vi "首页.vi"() -> ()   [LabVIEW 2016]
uses:
  <vilib>/Utility/miscctls.llb/LVPointTypeDef.ctl
  <vilib>/Utility/sysdir.llb/System Directory Type.ctl
  <vilib>/addons/database/_DB Variant To Data/Database Variant To Data.xnode
panel:
  out "显示":T1
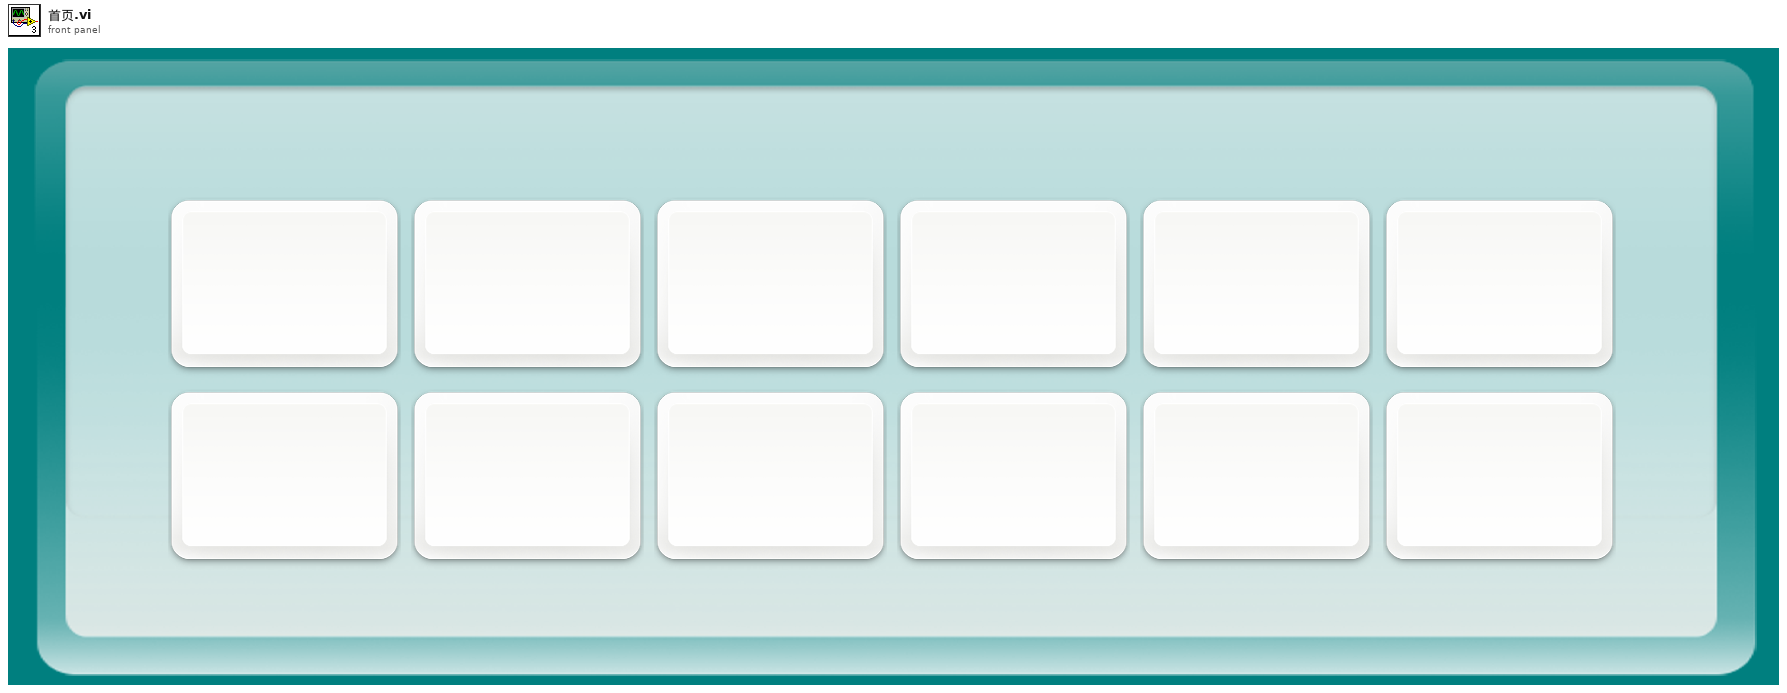
[diagram p1: front panel]
types:
  T1 = typedef "多数值显示.ctl" = cluster{"显示":T2, "显示 2":T2, "显示 3":T2, "显示 4":T2, "显示 5":T2, "显示 6":T2, "显示 12":T2, "显示 11":T2, "显示 10":T2, "显示 9":T2, "显示 8":T2, "显示 7":T2}
  T2 = typedef "数值显示.ctl" = cluster{"中文项目名称":string, "英文项目名称":string, "浓度":string, "单位":string}
  T3 = typedef "LVPointTypeDef.ctl" = cluster{"Horizontal":i16, "Vertical":i16}
  T4 = cluster{"显示参数中文名":string, "显示参数英文名":string, "显示浓度":string, "显示单位":string}[]
  T5 = cluster{"显示参数中文名":string, "显示参数英文名":string, "显示浓度":string, "显示单位":string}
  T6 = typedef "System Directory Type.ctl" = i32
  T7 = cluster{"AD0":dbl, "AD1":dbl, "AD2":dbl, "AD3":dbl, "AD4":dbl, "AD5":dbl, "AD6":dbl, "AD7":dbl}
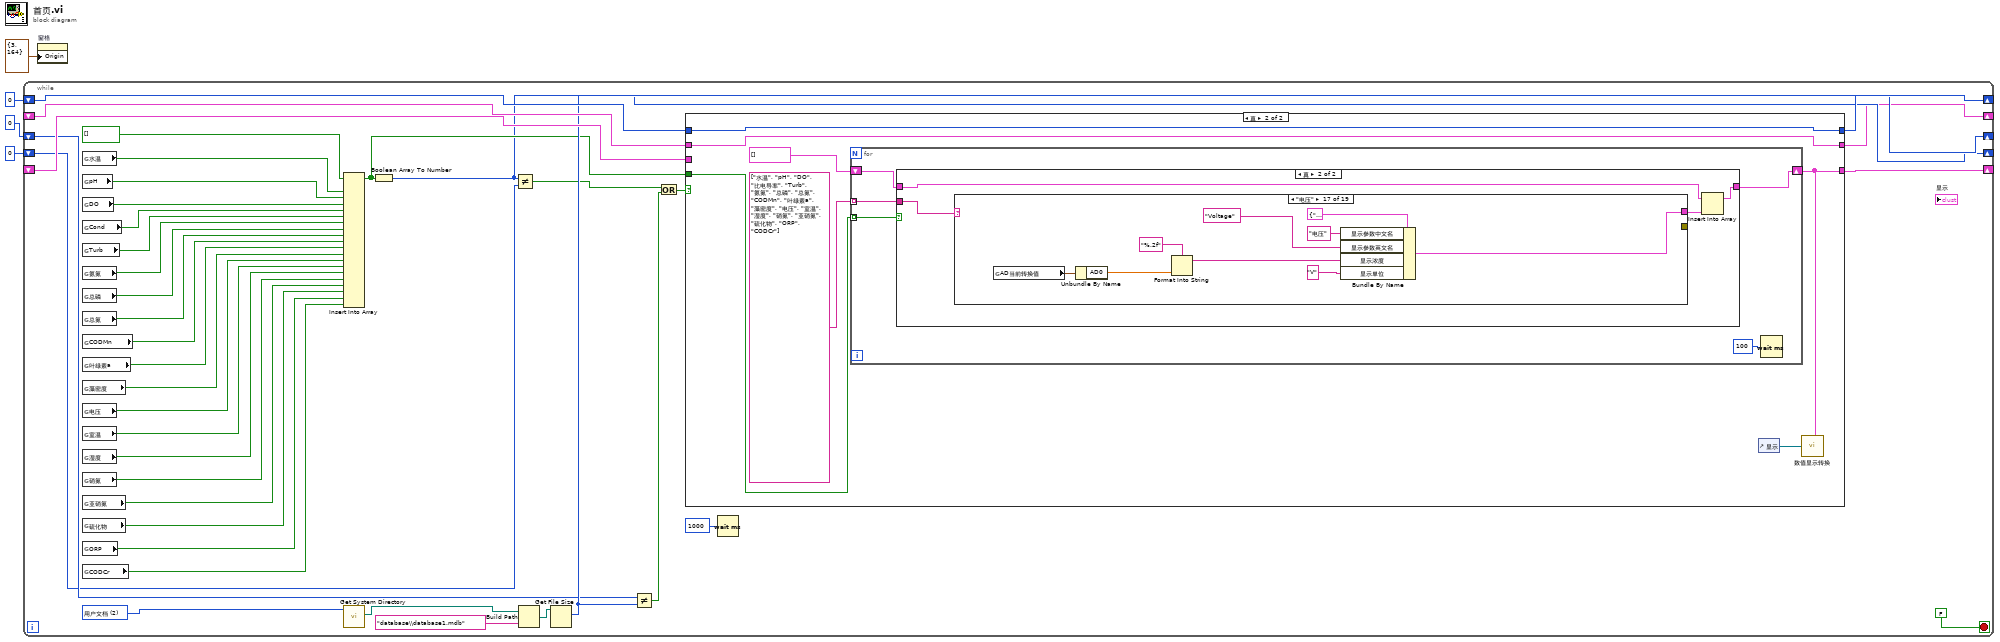
[diagram p0: block diagram]
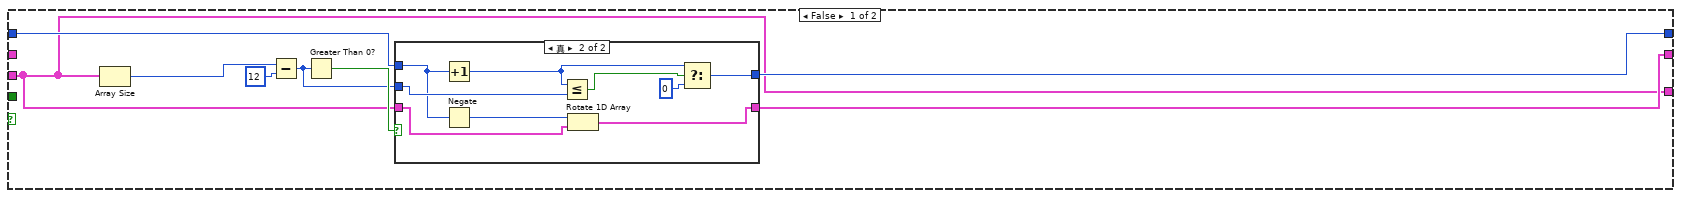
[diagram p2: hidden frame]
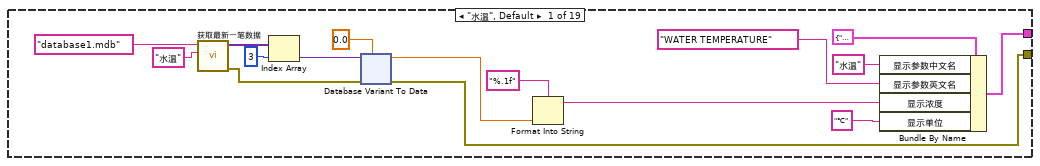
[diagram p5: hidden frame]
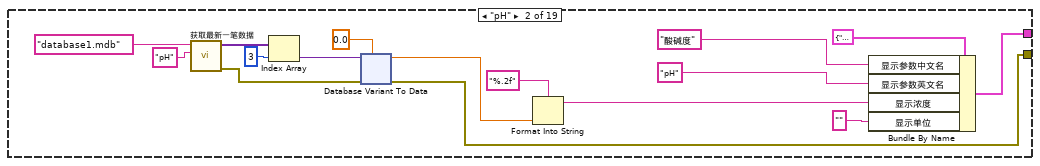
[diagram p6: hidden frame]
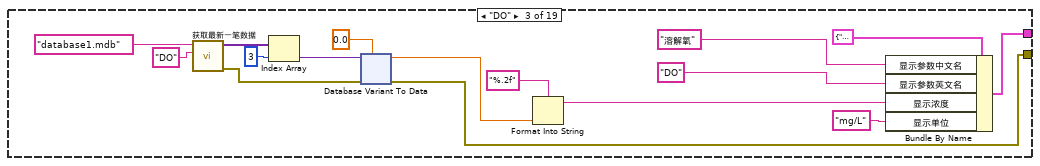
[diagram p7: hidden frame]
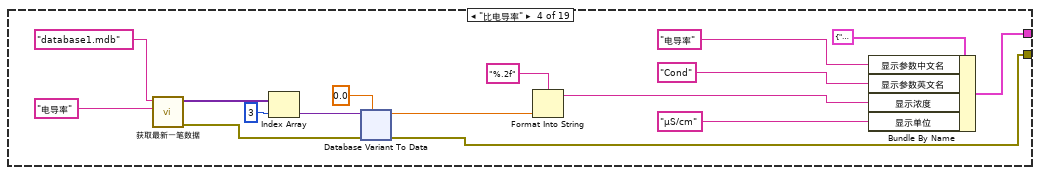
[diagram p8: hidden frame]
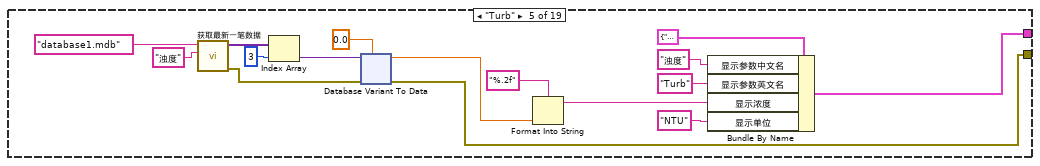
[diagram p9: hidden frame]
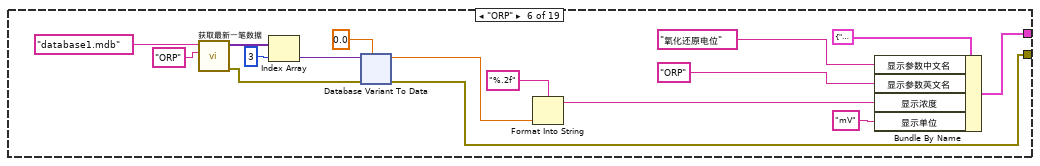
[diagram p10: hidden frame]
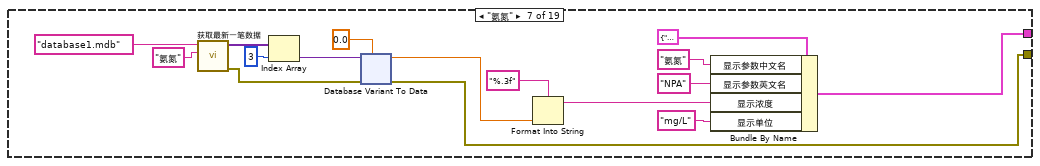
[diagram p11: hidden frame]
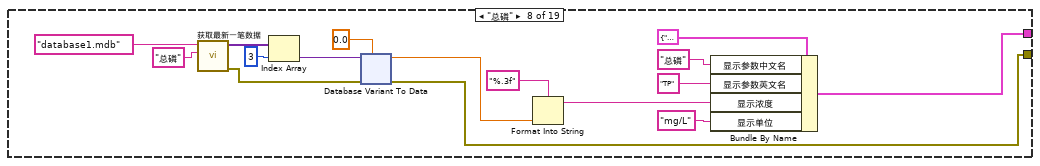
[diagram p12: hidden frame]
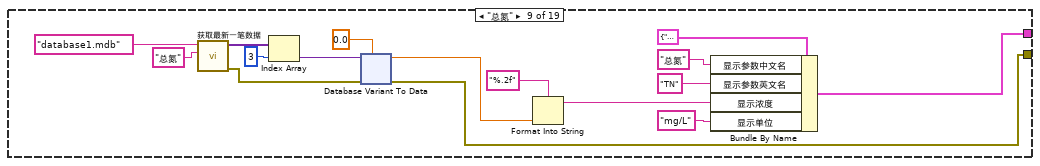
[diagram p13: hidden frame]
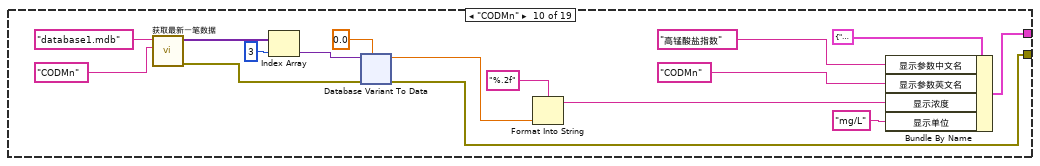
[diagram p14: hidden frame]
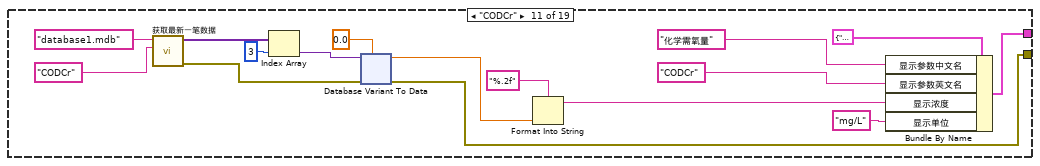
[diagram p15: hidden frame]
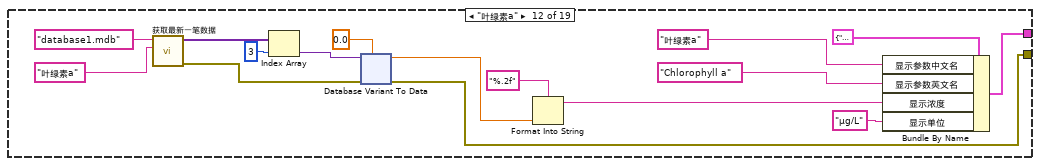
[diagram p16: hidden frame]
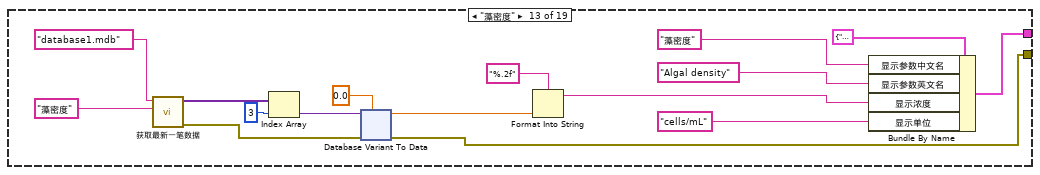
[diagram p17: hidden frame]
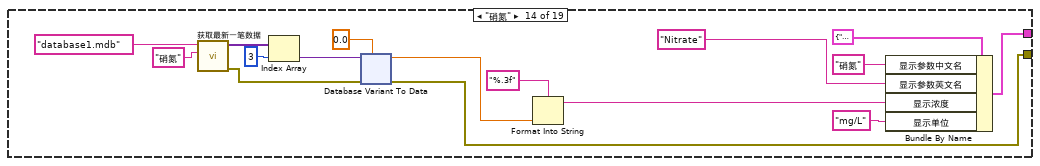
[diagram p18: hidden frame]
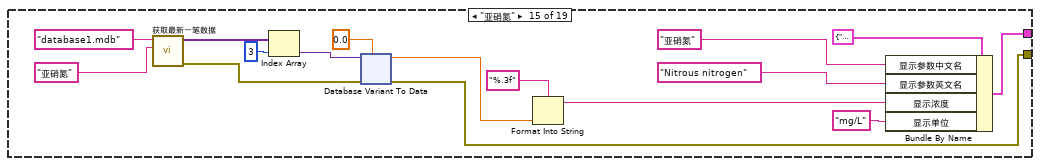
[diagram p19: hidden frame]
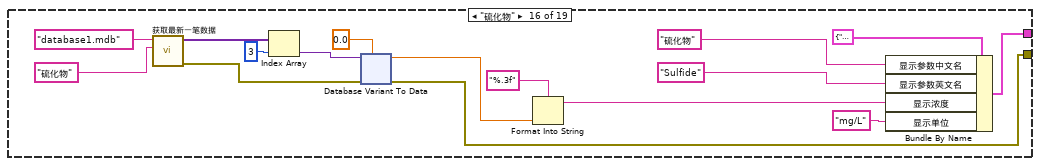
[diagram p20: hidden frame]
diagram:
  n1 = while {
    shift-right: [w42] -> _
    shift-left: _ -> [w41]
    shift-right: [w40] -> _
    shift-left: 0 -> [w43]
    shift-right: [w5] -> _
    shift-left: _ -> [w39]
    shift-right: [w34] -> _
    shift-left: i64 0 ("size (in bytes)") -> [w33]
    shift-right: [w12] -> _
    shift-left: u32 0 -> [w11]
    stop <- FALSE stop-if-true
    w38 = T6 2 items=["用户目录"=0, "用户桌面"=1, "用户文档"=2, "用户应用程序数据"=3, "用户设置"=4, "用户临时目录"=5, "公共文档"=6, "公共应用程序数据"=7, "公共设置"=8, "公共缓存"=13, "系统核心库"=9, "系统安装库"=10, "应用程序文件"=11, "启动盘根目录"=12] ("system directory type")
    n2 = global read "首页设置全局变量.vi" "水温"() -> (w26:bool)
    n3 = global read "首页设置全局变量.vi" "pH"() -> (w25:bool)
    n4 = global read "首页设置全局变量.vi" "DO"() -> (w24:bool)
    n5 = global read "首页设置全局变量.vi" "Cond"() -> (w23:bool)
    n6 = global read "首页设置全局变量.vi" "Turb"() -> (w22:bool)
    n7 = global read "首页设置全局变量.vi" "氨氮"() -> (w21:bool)
    n8 = global read "首页设置全局变量.vi" "总磷"() -> (w20:bool)
    n9 = global read "首页设置全局变量.vi" "总氮"() -> (w19:bool)
    n10 = global read "首页设置全局变量.vi" "CODMn"() -> (w18:bool)
    n11 = global read "首页设置全局变量.vi" "叶绿素a"() -> (w17:bool)
    n12 = global read "首页设置全局变量.vi" "藻密度"() -> (w16:bool)
    n13 = global read "首页设置全局变量.vi" "电压"() -> (w15:bool)
    n14 = global read "首页设置全局变量.vi" "室温"() -> (w14:bool)
    n15 = global read "首页设置全局变量.vi" "湿度"() -> (w28:bool)
    n16 = global read "首页设置全局变量.vi" "硝氮"() -> (w29:bool)
    n17 = global read "首页设置全局变量.vi" "亚硝氮"() -> (w30:bool)
    n18 = global read "首页设置全局变量.vi" "硫化物"() -> (w31:bool)
    n19 = global read "首页设置全局变量.vi" "ORP"() -> (w32:bool)
    n20 = global read "首页设置全局变量.vi" "CODCr"() -> (w6:bool)
    n21 = Insert Into Array(array=bool[] [], new element #1=w26, new element #2=w25, new element #3=w24, new element #4=w23, new element #5=w22, new element #6=w21, new element #7=w20, new element #8=w19, new element #9=w18, new element #10=w17, new element #11=w16, new element #12=w15, new element #13=w14, new element #14=w28, new element #15=w29, new element #16=w30, new element #17=w31, new element #18=w32, new element #19=w6) -> (w13:bool[])  [unwired: 1 in]
    n22 = call <vilib>:"Get System Directory.vi"("system directory type"=w38) -> ("system directory"=w37:path)  [unwired: 10 in]
    n23 = Boolean Array To Number(Boolean array=w13) -> (number=w12:u32)
    n24 = Not Equal?(x=w12, y=w11) -> (x != y?=w10:bool)
    n25 = Build Path(base path=w37, name or relative path="database\\database1.mdb" ("名称或相对路径")) -> (appended path=w35:path)
    n26 = Get File Size(file=w35) -> (size (in bytes)=w34:i64)  [unwired: 1 in, 2 out]
    n27 = Not Equal?(x=w33, y=w34) -> (x != y?=w9:bool)
    n28 = Or(x=w10, y=w9) -> (x .or. y?=w8:bool)
    n29 = case shown="真" w8 {
      tunnel: w43 -> [w52 w67]
      tunnel: [w45 w63] -> w42
      tunnel: w41 -> [w45 _]
      tunnel: [w51 w67] -> w40
      tunnel: [w46 w66] -> w5
      tunnel: w39 -> [_ w66]
      tunnel: w13 -> [_ w65]
      frame False {
        n30 = Array Size(array=w45) -> (size(s)=w50:i32)
        n31 = Subtract(x=w50, y=12) -> (x-y=w47:i32)
        n32 = Greater Than 0?(x=w47) -> (x > 0?=w48:bool)
        n33 = case shown="真" w48 {
          tunnel: w45 -> [w53 w62]
          tunnel: w52 -> [_ w55]
          tunnel: [w53 w61] -> w46
          tunnel: [_ w56] -> w51
          tunnel: w47 -> [_ w59]
          frame False {
          }
          frame True {
            n34 = Increment(x=w55) -> (x+1=w60:i32)
            n35 = Negate(x=w55) -> (-x=w54:i32)
            n36 = Less Or Equal?(x=w60, y=w59) -> (x <= y?=w58:bool)
            n37 = Rotate 1D Array(1:w62, 2:w54) -> (0:w61:T4)
            n38 = Select(t=w60, s=w58, f=0) -> (s? t:f=w56:i32)
          }
        }
      }
      frame True {
        n39 = for {
          tunnel: w65 -> [w74] mode=indexing
          tunnel: string[] ["水温", "pH", "DO", "比电导率", "Turb", "氨氮", "总磷", "总氮", "CODMn", "叶绿素a", "藻密度", "电压", "室温", "湿度", "硝氮", "亚硝氮", "硫化物", "ORP", "CODCr"] -> [w73] mode=indexing
          shift-right: [w71] -> w63
          shift-left: T4 [] -> [w72]
          n40 = case shown="真" w74 {
            tunnel: w73 -> [_ w79]
            tunnel: w72 -> [w75 w78]
            tunnel: [w75 w77] -> w71
            frame False {
            }
            frame True {
              n41 = case shown="\"电压\"" w79 {
                tunnel: [w89 w139 w187 w235 w283 w331 w379 w427 w475 w523 w571 w619 w667 w715 w763 w811 w852 w861 w870] -> w76
                tunnel: [w88 w136 w184 w231 w279 w327 w368 w416 w464 w512 w560 w615 w656 w704 w752 w800 _ _ _] -> _
                frame "水温", Default {
                  n42 = call "获取最新一笔数据.vi"("table"="水温", "database"="database1.mdb" ("名称或相对路径")) -> ("error out"=w80:errorcluster, "子数组"=w85:variant[])  [unwired: 8 in]
                  n43 = Index Array(array=w85, index=3 ("索引")) -> (element=w83:variant)
                  n44 = xnode "Database Variant To Data"("database variant"=w83, "error in (no error)"=w80, "type"=0.0) -> ("data"=w87:dbl, "error out"=w88:errorcluster)
                  n45 = Format Into String(format string="%.1f" ("格式字符串"), w87) -> (resulting string=w90:string)  [unwired: 2 in, 1 out]
                  n46 = Bundle By Name(cluster=T5 {"显示参数中文名"="", "显示参数英文名"="", "显示浓度"="", "显示单位"=""} ("元素"), "显示参数中文名"="水温", "显示参数英文名"="WATER TEMPERATURE", "显示浓度"=w90, "显示单位"="℃") -> (w89:T5)
                }
                frame "pH" {
                  n47 = call "获取最新一笔数据.vi"("table"="pH", "database"="database1.mdb" ("名称或相对路径")) -> ("error out"=w128:errorcluster, "子数组"=w133:variant[])  [unwired: 8 in]
                  n48 = Index Array(array=w133, index=3 ("索引")) -> (element=w131:variant)
                  n49 = xnode "Database Variant To Data"("database variant"=w131, "error in (no error)"=w128, "type"=0.0) -> ("data"=w135:dbl, "error out"=w136:errorcluster)
                  n50 = Format Into String(format string="%.2f" ("格式字符串"), w135) -> (resulting string=w137:string)  [unwired: 2 in, 1 out]
                  n51 = Bundle By Name(cluster=T5 {"显示参数中文名"="", "显示参数英文名"="", "显示浓度"="", "显示单位"=""} ("元素"), "显示参数中文名"="酸碱度", "显示参数英文名"="pH", "显示浓度"=w137, "显示单位"="") -> (w139:T5)
                }
                frame "DO" {
                  n52 = call "获取最新一笔数据.vi"("table"="DO", "database"="database1.mdb" ("名称或相对路径")) -> ("error out"=w176:errorcluster, "子数组"=w181:variant[])  [unwired: 8 in]
                  n53 = Index Array(array=w181, index=3 ("索引")) -> (element=w179:variant)
                  n54 = xnode "Database Variant To Data"("database variant"=w179, "error in (no error)"=w176, "type"=0.0) -> ("data"=w183:dbl, "error out"=w184:errorcluster)
                  n55 = Format Into String(format string="%.2f" ("格式字符串"), w183) -> (resulting string=w185:string)  [unwired: 2 in, 1 out]
                  n56 = Bundle By Name(cluster=T5 {"显示参数中文名"="", "显示参数英文名"="", "显示浓度"="", "显示单位"=""} ("元素"), "显示参数中文名"="溶解氧", "显示参数英文名"="DO", "显示浓度"=w185, "显示单位"="mg/L") -> (w187:T5)
                }
                frame "比电导率" {
                  n57 = call "获取最新一笔数据.vi"("table"="电导率", "database"="database1.mdb" ("名称或相对路径")) -> ("error out"=w224:errorcluster, "子数组"=w229:variant[])  [unwired: 8 in]
                  n58 = Index Array(array=w229, index=3 ("索引")) -> (element=w227:variant)
                  n59 = xnode "Database Variant To Data"("database variant"=w227, "error in (no error)"=w224, "type"=0.0) -> ("data"=w232:dbl, "error out"=w231:errorcluster)
                  n60 = Format Into String(format string="%.2f" ("格式字符串"), w232) -> (resulting string=w233:string)  [unwired: 2 in, 1 out]
                  n61 = Bundle By Name(cluster=T5 {"显示参数中文名"="", "显示参数英文名"="", "显示浓度"="", "显示单位"=""} ("元素"), "显示参数中文名"="电导率", "显示参数英文名"="Cond", "显示浓度"=w233, "显示单位"="μS/cm") -> (w235:T5)
                }
                frame "Turb" {
                  n62 = call "获取最新一笔数据.vi"("table"="浊度", "database"="database1.mdb" ("名称或相对路径")) -> ("error out"=w272:errorcluster, "子数组"=w277:variant[])  [unwired: 8 in]
                  n63 = Index Array(array=w277, index=3 ("索引")) -> (element=w275:variant)
                  n64 = xnode "Database Variant To Data"("database variant"=w275, "error in (no error)"=w272, "type"=0.0) -> ("data"=w280:dbl, "error out"=w279:errorcluster)
                  n65 = Format Into String(format string="%.2f" ("格式字符串"), w280) -> (resulting string=w281:string)  [unwired: 2 in, 1 out]
                  n66 = Bundle By Name(cluster=T5 {"显示参数中文名"="", "显示参数英文名"="", "显示浓度"="", "显示单位"=""} ("元素"), "显示参数中文名"="浊度", "显示参数英文名"="Turb", "显示浓度"=w281, "显示单位"="NTU") -> (w283:T5)
                }
                frame "ORP" {
                  n67 = call "获取最新一笔数据.vi"("table"="ORP", "database"="database1.mdb" ("名称或相对路径")) -> ("error out"=w320:errorcluster, "子数组"=w325:variant[])  [unwired: 8 in]
                  n68 = Index Array(array=w325, index=3 ("索引")) -> (element=w323:variant)
                  n69 = xnode "Database Variant To Data"("database variant"=w323, "error in (no error)"=w320, "type"=0.0) -> ("data"=w328:dbl, "error out"=w327:errorcluster)
                  n70 = Format Into String(format string="%.2f" ("格式字符串"), w328) -> (resulting string=w329:string)  [unwired: 2 in, 1 out]
                  n71 = Bundle By Name(cluster=T5 {"显示参数中文名"="", "显示参数英文名"="", "显示浓度"="", "显示单位"=""} ("元素"), "显示参数中文名"="氧化还原电位", "显示参数英文名"="ORP", "显示浓度"=w329, "显示单位"="mV") -> (w331:T5)
                }
                frame "氨氮" {
                  n72 = call "获取最新一笔数据.vi"("table"="氨氮", "database"="database1.mdb" ("名称或相对路径")) -> ("error out"=w369:errorcluster, "子数组"=w375:variant[])  [unwired: 8 in]
                  n73 = Index Array(array=w375, index=3 ("索引")) -> (element=w373:variant)
                  n74 = xnode "Database Variant To Data"("database variant"=w373, "error in (no error)"=w369, "type"=0.0) -> ("data"=w370:dbl, "error out"=w368:errorcluster)
                  n75 = Format Into String(format string="%.3f" ("格式字符串"), w370) -> (resulting string=w377:string)  [unwired: 2 in, 1 out]
                  n76 = Bundle By Name(cluster=T5 {"显示参数中文名"="", "显示参数英文名"="", "显示浓度"="", "显示单位"=""} ("元素"), "显示参数中文名"="氨氮", "显示参数英文名"="NPA", "显示浓度"=w377, "显示单位"="mg/L") -> (w379:T5)
                }
                frame "总磷" {
                  n77 = call "获取最新一笔数据.vi"("table"="总磷", "database"="database1.mdb" ("名称或相对路径")) -> ("error out"=w417:errorcluster, "子数组"=w423:variant[])  [unwired: 8 in]
                  n78 = Index Array(array=w423, index=3 ("索引")) -> (element=w421:variant)
                  n79 = xnode "Database Variant To Data"("database variant"=w421, "error in (no error)"=w417, "type"=0.0) -> ("data"=w418:dbl, "error out"=w416:errorcluster)
                  n80 = Format Into String(format string="%.3f" ("格式字符串"), w418) -> (resulting string=w425:string)  [unwired: 2 in, 1 out]
                  n81 = Bundle By Name(cluster=T5 {"显示参数中文名"="", "显示参数英文名"="", "显示浓度"="", "显示单位"=""} ("元素"), "显示参数中文名"="总磷", "显示参数英文名"="TP", "显示浓度"=w425, "显示单位"="mg/L") -> (w427:T5)
                }
                frame "总氮" {
                  n82 = call "获取最新一笔数据.vi"("table"="总氮", "database"="database1.mdb" ("名称或相对路径")) -> ("error out"=w465:errorcluster, "子数组"=w471:variant[])  [unwired: 8 in]
                  n83 = Index Array(array=w471, index=3 ("索引")) -> (element=w469:variant)
                  n84 = xnode "Database Variant To Data"("database variant"=w469, "error in (no error)"=w465, "type"=0.0) -> ("data"=w466:dbl, "error out"=w464:errorcluster)
                  n85 = Format Into String(format string="%.2f" ("格式字符串"), w466) -> (resulting string=w473:string)  [unwired: 2 in, 1 out]
                  n86 = Bundle By Name(cluster=T5 {"显示参数中文名"="", "显示参数英文名"="", "显示浓度"="", "显示单位"=""} ("元素"), "显示参数中文名"="总氮", "显示参数英文名"="TN", "显示浓度"=w473, "显示单位"="mg/L") -> (w475:T5)
                }
                frame "CODMn" {
                  n87 = call "获取最新一笔数据.vi"("table"="CODMn", "database"="database1.mdb" ("名称或相对路径")) -> ("error out"=w513:errorcluster, "子数组"=w519:variant[])  [unwired: 8 in]
                  n88 = Index Array(array=w519, index=3 ("索引")) -> (element=w517:variant)
                  n89 = xnode "Database Variant To Data"("database variant"=w517, "error in (no error)"=w513, "type"=0.0) -> ("data"=w514:dbl, "error out"=w512:errorcluster)
                  n90 = Format Into String(format string="%.2f" ("格式字符串"), w514) -> (resulting string=w521:string)  [unwired: 2 in, 1 out]
                  n91 = Bundle By Name(cluster=T5 {"显示参数中文名"="", "显示参数英文名"="", "显示浓度"="", "显示单位"=""} ("元素"), "显示参数中文名"="高锰酸盐指数", "显示参数英文名"="CODMn", "显示浓度"=w521, "显示单位"="mg/L") -> (w523:T5)
                }
                frame "CODCr" {
                  n92 = call "获取最新一笔数据.vi"("table"="CODCr", "database"="database1.mdb" ("名称或相对路径")) -> ("error out"=w561:errorcluster, "子数组"=w567:variant[])  [unwired: 8 in]
                  n93 = Index Array(array=w567, index=3 ("索引")) -> (element=w565:variant)
                  n94 = xnode "Database Variant To Data"("database variant"=w565, "error in (no error)"=w561, "type"=0.0) -> ("data"=w562:dbl, "error out"=w560:errorcluster)
                  n95 = Format Into String(format string="%.2f" ("格式字符串"), w562) -> (resulting string=w569:string)  [unwired: 2 in, 1 out]
                  n96 = Bundle By Name(cluster=T5 {"显示参数中文名"="", "显示参数英文名"="", "显示浓度"="", "显示单位"=""} ("元素"), "显示参数中文名"="化学需氧量", "显示参数英文名"="CODCr", "显示浓度"=w569, "显示单位"="mg/L") -> (w571:T5)
                }
                frame "叶绿素a" {
                  n97 = call "获取最新一笔数据.vi"("table"="叶绿素a", "database"="database1.mdb" ("名称或相对路径")) -> ("error out"=w608:errorcluster, "子数组"=w613:variant[])  [unwired: 8 in]
                  n98 = Index Array(array=w613, index=3 ("索引")) -> (element=w611:variant)
                  n99 = xnode "Database Variant To Data"("database variant"=w611, "error in (no error)"=w608, "type"=0.0) -> ("data"=w616:dbl, "error out"=w615:errorcluster)
                  n100 = Format Into String(format string="%.2f" ("格式字符串"), w616) -> (resulting string=w617:string)  [unwired: 2 in, 1 out]
                  n101 = Bundle By Name(cluster=T5 {"显示参数中文名"="", "显示参数英文名"="", "显示浓度"="", "显示单位"=""} ("元素"), "显示参数中文名"="叶绿素a", "显示参数英文名"="Chlorophyll a", "显示浓度"=w617, "显示单位"="μg/L") -> (w619:T5)
                }
                frame "藻密度" {
                  n102 = call "获取最新一笔数据.vi"("table"="藻密度", "database"="database1.mdb" ("名称或相对路径")) -> ("error out"=w657:errorcluster, "子数组"=w663:variant[])  [unwired: 8 in]
                  n103 = Index Array(array=w663, index=3 ("索引")) -> (element=w661:variant)
                  n104 = xnode "Database Variant To Data"("database variant"=w661, "error in (no error)"=w657, "type"=0.0) -> ("data"=w658:dbl, "error out"=w656:errorcluster)
                  n105 = Format Into String(format string="%.2f" ("格式字符串"), w658) -> (resulting string=w665:string)  [unwired: 2 in, 1 out]
                  n106 = Bundle By Name(cluster=T5 {"显示参数中文名"="", "显示参数英文名"="", "显示浓度"="", "显示单位"=""} ("元素"), "显示参数中文名"="藻密度", "显示参数英文名"="Algal density", "显示浓度"=w665, "显示单位"="cells/mL") -> (w667:T5)
                }
                frame "硝氮" {
                  n107 = call "获取最新一笔数据.vi"("table"="硝氮", "database"="database1.mdb" ("名称或相对路径")) -> ("error out"=w705:errorcluster, "子数组"=w711:variant[])  [unwired: 8 in]
                  n108 = Index Array(array=w711, index=3 ("索引")) -> (element=w709:variant)
                  n109 = xnode "Database Variant To Data"("database variant"=w709, "error in (no error)"=w705, "type"=0.0) -> ("data"=w706:dbl, "error out"=w704:errorcluster)
                  n110 = Format Into String(format string="%.3f" ("格式字符串"), w706) -> (resulting string=w713:string)  [unwired: 2 in, 1 out]
                  n111 = Bundle By Name(cluster=T5 {"显示参数中文名"="", "显示参数英文名"="", "显示浓度"="", "显示单位"=""} ("元素"), "显示参数中文名"="硝氮", "显示参数英文名"="Nitrate", "显示浓度"=w713, "显示单位"="mg/L") -> (w715:T5)
                }
                frame "亚硝氮" {
                  n112 = call "获取最新一笔数据.vi"("table"="亚硝氮", "database"="database1.mdb" ("名称或相对路径")) -> ("error out"=w753:errorcluster, "子数组"=w759:variant[])  [unwired: 8 in]
                  n113 = Index Array(array=w759, index=3 ("索引")) -> (element=w757:variant)
                  n114 = xnode "Database Variant To Data"("database variant"=w757, "error in (no error)"=w753, "type"=0.0) -> ("data"=w754:dbl, "error out"=w752:errorcluster)
                  n115 = Format Into String(format string="%.3f" ("格式字符串"), w754) -> (resulting string=w761:string)  [unwired: 2 in, 1 out]
                  n116 = Bundle By Name(cluster=T5 {"显示参数中文名"="", "显示参数英文名"="", "显示浓度"="", "显示单位"=""} ("元素"), "显示参数中文名"="亚硝氮", "显示参数英文名"="Nitrous nitrogen", "显示浓度"=w761, "显示单位"="mg/L") -> (w763:T5)
                }
                frame "硫化物" {
                  n117 = call "获取最新一笔数据.vi"("table"="硫化物", "database"="database1.mdb" ("名称或相对路径")) -> ("error out"=w801:errorcluster, "子数组"=w807:variant[])  [unwired: 8 in]
                  n118 = Index Array(array=w807, index=3 ("索引")) -> (element=w805:variant)
                  n119 = xnode "Database Variant To Data"("database variant"=w805, "error in (no error)"=w801, "type"=0.0) -> ("data"=w802:dbl, "error out"=w800:errorcluster)
                  n120 = Format Into String(format string="%.3f" ("格式字符串"), w802) -> (resulting string=w809:string)  [unwired: 2 in, 1 out]
                  n121 = Bundle By Name(cluster=T5 {"显示参数中文名"="", "显示参数英文名"="", "显示浓度"="", "显示单位"=""} ("元素"), "显示参数中文名"="硫化物", "显示参数英文名"="Sulfide", "显示浓度"=w809, "显示单位"="mg/L") -> (w811:T5)
                }
                frame "电压" {
                  n122 = global read "断电保存全局变量.vi" "AD当前转换值"() -> (w849:T7)
                  n123 = Unbundle By Name(w849) -> ("AD0"=w848:dbl)
                  n124 = Format Into String(format string="%.2f" ("格式字符串"), w848) -> (resulting string=w850:string)  [unwired: 2 in, 1 out]
                  n125 = Bundle By Name(cluster=T5 {"显示参数中文名"="", "显示参数英文名"="", "显示浓度"="", "显示单位"=""} ("元素"), "显示参数中文名"="电压", "显示参数英文名"="Voltage", "显示浓度"=w850, "显示单位"="V") -> (w852:T5)
                }
                frame "室温" {
                  n126 = global read "断电保存全局变量.vi" "AD当前转换值"() -> (w858:T7)
                  n127 = Unbundle By Name(w858) -> ("AD4"=w857:dbl)
                  n128 = Format Into String(format string="%.2f" ("格式字符串"), w857) -> (resulting string=w859:string)  [unwired: 2 in, 1 out]
                  n129 = Bundle By Name(cluster=T5 {"显示参数中文名"="", "显示参数英文名"="", "显示浓度"="", "显示单位"=""} ("元素"), "显示参数中文名"="室温", "显示参数英文名"="Room temperature", "显示浓度"=w859, "显示单位"="℃") -> (w861:T5)
                }
                frame "湿度" {
                  n130 = global read "断电保存全局变量.vi" "AD当前转换值"() -> (w867:T7)
                  n131 = Unbundle By Name(w867) -> ("AD5"=w866:dbl)
                  n132 = Format Into String(format string="%.2f" ("格式字符串"), w866) -> (resulting string=w868:string)  [unwired: 2 in, 1 out]
                  n133 = Bundle By Name(cluster=T5 {"显示参数中文名"="", "显示参数英文名"="", "显示浓度"="", "显示单位"=""} ("元素"), "显示参数中文名"="湿度", "显示参数英文名"="humidity", "显示浓度"=w868, "显示单位"="%RH") -> (w870:T5)
                }
              }
              n134 = Insert Into Array(array=w78, new element=w76) -> (w77:T4)  [unwired: 1 in]
            }
          }
          n135 = Wait (ms)(milliseconds to wait=u32 100 ("等待时间（毫秒）")) -> ()  [unwired: 1 out]
        }
        n136 = control-ref of="显示"() -> (w64:refnum<vi>)
        n137 = call "数值显示转换.vi"("显示"=w64, "数组"=w63) -> ()  [unwired: 10 in]
      }
    }
    n138 = Wait (ms)(milliseconds to wait=u32 1000 ("等待时间（毫秒）")) -> ()  [unwired: 1 out]
  }
  n139 = property on="窗格" class="Pane"("Origin"=T3 {"Horizontal"=3, "Vertical"=164} ("原点")) -> ()  [unwired: 2 in, 2 out]
